vi "Get Transfer UIs.vi"(8 "error in (no error)":errorcluster, 11 "Component UI in":refnum<class "UDPlog User Interfaces.lvclass">) -> (0 "error out":errorcluster, 1 "Tx Transfer UI":refnum<class "User Interface.lvclass">, 2 "Rx Transfer UI":refnum<class "User Interface.lvclass">, 3 "Component UI out":refnum<class "UDPlog User Interfaces.lvclass">)   [LabVIEW 2023, in "UDPlog.lvlib" / "UDPlog User Interfaces.lvclass"]
uses:
  UDPlog User Interfaces.lvclass
  Users/Public/Documents/National Instruments/NI VeriStand 2023/Custom Devices/Data Sharing Framework/Linux_x64/DSF Core.lvlibp/Classes/User Interface/User Interface.lvclass
  Transfer Tx/UDPlog Transfer Tx User Interface.lvclass
  C:/Users/Public/Documents/National Instruments/NI VeriStand 2023/Custom Devices/Data Sharing Framework/Linux_x64/DSF Core.lvlibp/Classes/User Interface/User Interface.lvclass
  Transfer Rx/UDPlog Transfer Rx User Interface.lvclass
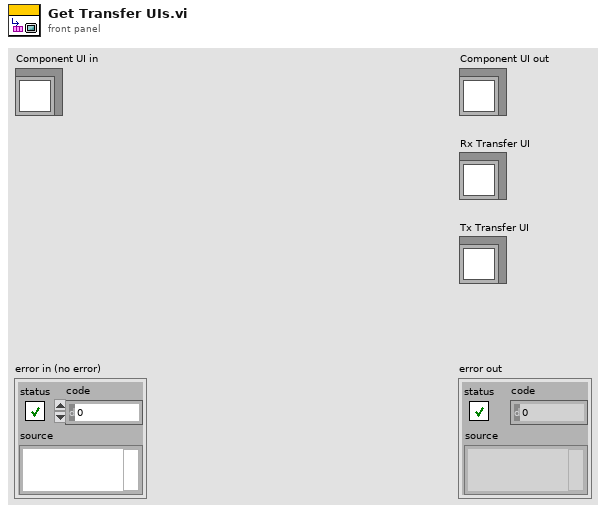
[diagram p1: front panel]
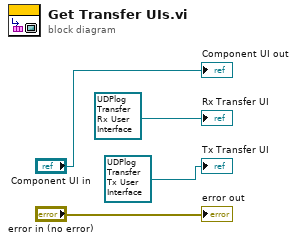
[diagram p0: block diagram]
diagram:
  "error out" <- "error in (no error)"
  "Component UI out" <- "Component UI in"
  "Rx Transfer UI" <- refnum<class "UDPlog Transfer Rx User Interface.lvclass"> refnum ("UDPlog.lvlib:UDPlog Transfer Rx User Interface.lvclass")
  "Tx Transfer UI" <- refnum<class "UDPlog Transfer Tx User Interface.lvclass"> refnum ("UDPlog.lvlib:UDPlog Transfer Tx User Interface.lvclass")
